vi "multimetr.vi"(1 "Zapytanie":string, 2 "Model [0-1]":u8 max=2 step=1, 3 "Jednostka [0-2]":u8 max=2 step=1, 4 "Rezystancja [DBL]":dbl) -> (0 "Ramka":string)   [LabVIEW 2020]
panel:
  out "Dlugosc":i32
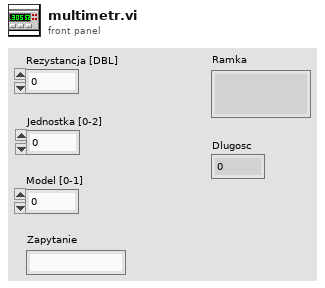
[diagram p1: front panel]
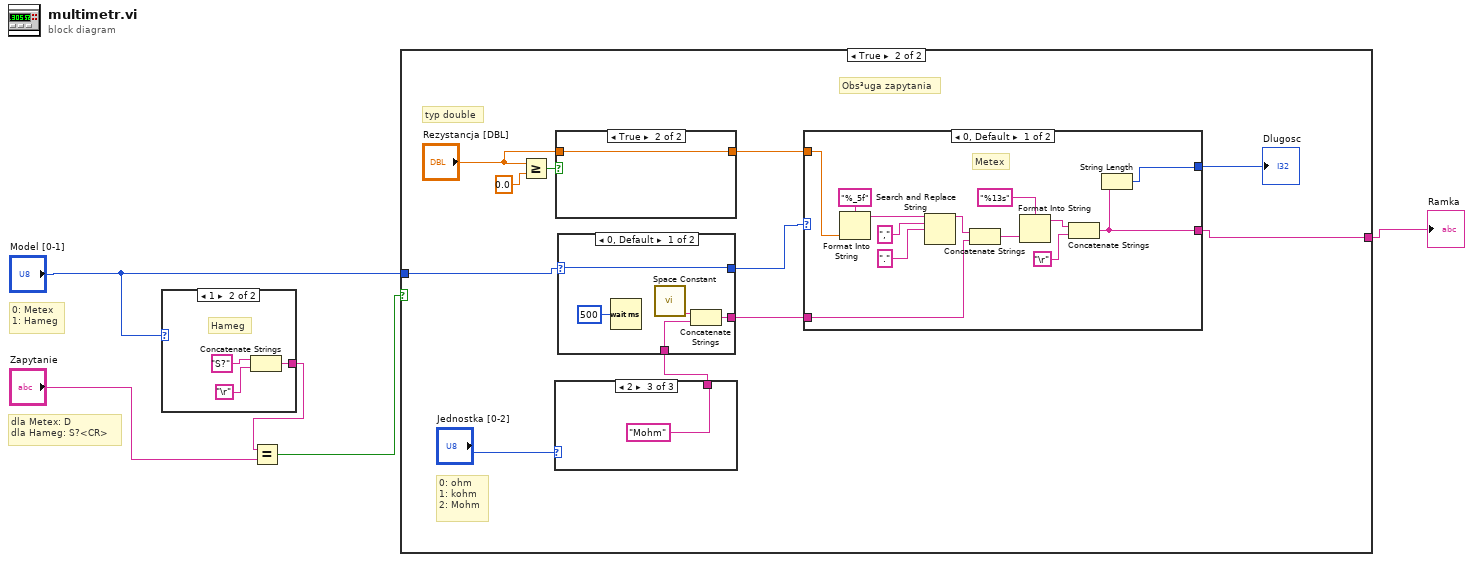
[diagram p0: block diagram]
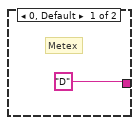
[diagram p2: hidden frame]
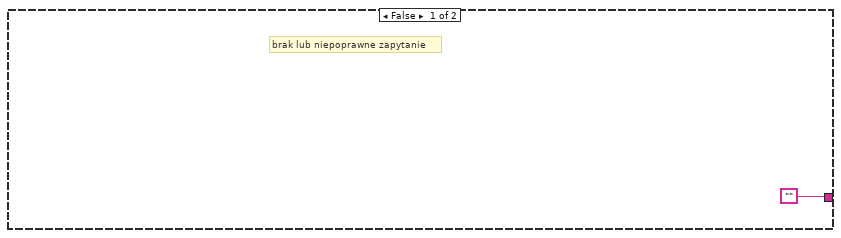
[diagram p3: hidden frame]
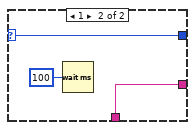
[diagram p4: hidden frame]
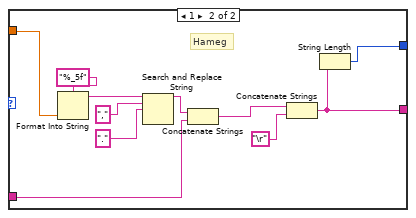
[diagram p5: hidden frame]
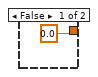
[diagram p6: hidden frame]
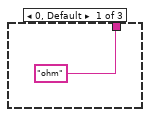
[diagram p7: hidden frame]
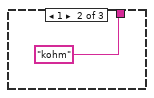
[diagram p8: hidden frame]
diagram:
  # "dla Metex: D\ndla Hameg: S?<CR>"
  # "0: Metex\n1: Hameg"
  n1 = case shown="1" "Model [0-1]" {
    tunnel: ["D" w7] -> w2
    frame 0, Default {
      # "Metex"
    }
    frame 1 {
      # "Hameg"
      n2 = Concatenate Strings("S?", "\r") -> (w7:string)
    }
  }
  n3 = Equal?(x=w2, y="Zapytanie") -> (x = y?=w1:bool)
  n4 = case shown="True" w1 {
    tunnel: "Model [0-1]" -> [_ w12]
    tunnel: ["" w11] -> w5
    frame False {
      # "brak lub niepoprawne zapytanie"
    }
    frame True {
      # "Obs³uga zapytania"
      # "typ double"
      # "0: ohm\n1: kohm\n2: Mohm"
      n5 = Greater Or Equal?(x="Rezystancja [DBL]", y=0.0) -> (x >= y?=w20:bool)
      n6 = case shown="2" "Jednostka [0-2]" {
        tunnel: ["ohm" "kohm" "Mohm"] -> w15
        frame 0, Default {
        }
        frame 1 {
        }
        frame 2 {
        }
      }
      n7 = case shown="True" w20 {
        tunnel: "Rezystancja [DBL]" -> [_ w55]
        tunnel: [0.0 w55] -> w17
        frame False {
        }
        frame True {
        }
      }
      n8 = case shown="0, Default" w12 {
        selector: w12 -> [w25 w29]
        tunnel: [w25 w29] -> w16
        tunnel: w15 -> [w23 w27]
        tunnel: [w24 w27] -> w14
        frame 0, Default {
          n9 = Wait (ms)(milliseconds to wait=u32 500) -> ()  [unwired: 1 out]
          n10 = call <vilib>:"Space Constant.vi"() -> ("String"=w22:string)
          n11 = Concatenate Strings(w22, w23) -> (w24:string)
        }
        frame 1 {
          n12 = Wait (ms)(milliseconds to wait=u32 100) -> ()  [unwired: 1 out]
        }
      }
      n13 = case shown="0, Default" w16 {
        tunnel: w17 -> [w41 w46]
        tunnel: w14 -> [w32 w47]
        tunnel: [w31 w44] -> w11
        tunnel: [w30 w43] -> w13
        frame 0, Default {
          # "Metex"
          n14 = Format Into String(format string="%_5f", w41) -> (resulting string=w36:string)  [unwired: 2 in, 1 out]
          n15 = Search and Replace String(input string=w36, search string=",", replace string="." ("replace string (\"\")")) -> (result string=w33:string)  [unwired: 5 in, 3 out]
          n16 = Concatenate Strings(w33, w32) -> (w39:string)
          n17 = Format Into String(format string="%13s", w39) -> (resulting string=w38:string)  [unwired: 2 in, 1 out]
          n18 = Concatenate Strings(w38, "\r") -> (w31:string)
          n19 = String Length(string=w31) -> (length=w30:i32)
        }
        frame 1 {
          # "Hameg"
          n20 = Format Into String(format string="%_5f", w46) -> (resulting string=w52:string)  [unwired: 2 in, 1 out]
          n21 = Search and Replace String(input string=w52, search string=",", replace string="." ("replace string (\"\")")) -> (result string=w53:string)  [unwired: 5 in, 3 out]
          n22 = Concatenate Strings(w53, w47) -> (w45:string)
          n23 = Concatenate Strings(w45, "\r") -> (w44:string)
          n24 = String Length(string=w44) -> (length=w43:i32)
        }
      }
      "Dlugosc" <- w13
    }
  }
  "Ramka" <- w5
